vi "PuTTY Connect.vi"   [LabVIEW 2020, in "NI_SFTP.lvlib"]
doc: "Connects to an SFTP server using the Plink executable typically installed with the PuTTY client."
uses:
  <vilib>/net/SFTP/NI_SFTP.lvlib
  <vilib>/net/SSH/Client/PuTTY/PuTTY Client.lvclass
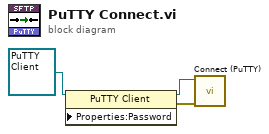
[diagram p0: block diagram]
diagram:
  n1 = property class="PuTTY Client" props=["Properties:Password"](reference=refnum<class "PuTTY Client.lvclass"> refnum ("NI_SSH.lvlib:PuTTY Client")) -> (reference out=w2:refnum<class "PuTTY Client.lvclass">, error out=w1:errorcluster)  [unwired: 2 in]
  n2 = call <vilib>:"Connect (PuTTY).vi"("error in"=w1, "client"=w2) -> ()  [unwired: 8 in, 2 out]
